vi "Motor Copy of Timer.vi"(1 "Command":enum16{"Start counting", "Read count", "Reset"}(ring)) -> (0 "Time out":dbl)   [LabVIEW 2010]
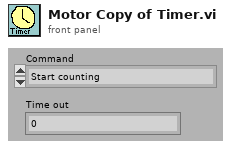
[diagram p1: front panel]
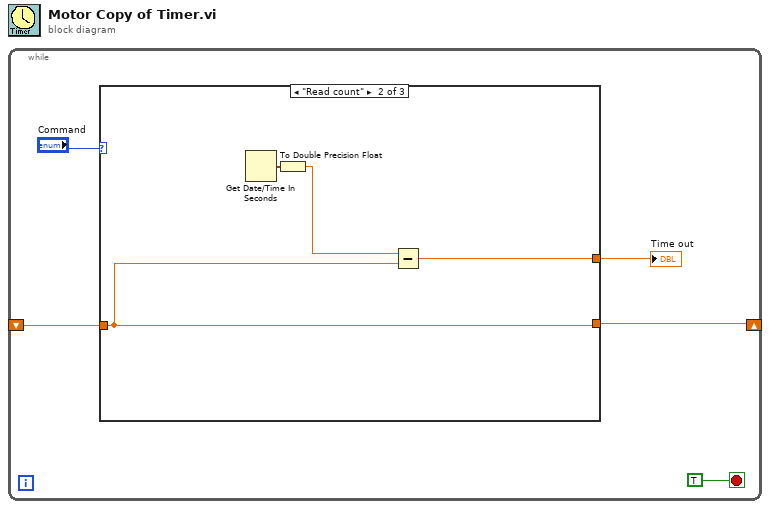
[diagram p0: block diagram]
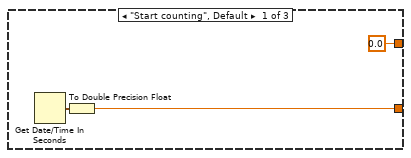
[diagram p2: hidden frame]
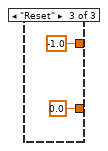
[diagram p3: hidden frame]
diagram:
  n1 = while {
    shift-right: [w2] -> _
    shift-left: _ -> [w4]
    stop <- TRUE stop-if-true
    n2 = case shown="\"Read count\"" "Command" {
      tunnel: w4 -> [_ w9 _]
      tunnel: [0.0 w10 -1.0] -> w3
      tunnel: [w6 w9 0.0] -> w2
      frame "Start counting", Default {
        n3 = Get Date/Time In Seconds() -> (seconds since 1Jan1904=w8:timestamp)
        n4 = To Double Precision Float(number=w8) -> (double precision float=w6:dbl)
      }
      frame "Read count" {
        n5 = Get Date/Time In Seconds() -> (seconds since 1Jan1904=w12:timestamp)
        n6 = To Double Precision Float(number=w12) -> (double precision float=w11:dbl)
        n7 = Subtract(x=w11, y=w9) -> (x-y=w10:dbl)
      }
      frame "Reset" {
      }
    }
    "Time out" <- w3
  }
